vi "PicoScope6000aSetupStreaming.vi"(0 "handle in":i16=16384, 1 "Streaming Acquisition Settings":T4={"preTriggerSamples"=0, "postTriggerSamples"=1000000, "Requested sampleInterval"=1.0, "sampleIntervalTimeUnits"=3} {"sampleIntervalTimeUnits" items=["femtoseconds", "picoseconds", "nanoseconds", "microseconds", "millseconds", "seconds"]; "postTriggerSamples" format="%_6p"; "preTriggerSamples" format="%_6p"}, 2 "Buffer and Transfer Settings":T3={"startIndex"=0, "Samples"=1000000, "Down Sample Ratio"=1, "Down-Sample Mode"=2147483648} {"Down-Sample Mode" items=["None"=2147483648, "Aggregate"=1, "Decimate"=2, "Average"=4]; "Down Sample Ratio" step=1; "Samples" format="%_6p"}, 3 "enabled array":i16[](array[numeric])=[1, 1, 0, 0, 0, 0, 0, 0, 0, 0], 7 "Data Pointers In":T1, 9 "Number of Buffers":i32=1, 11 "error in (no error)":errorcluster) -> (4 "handle out":i16=16384, 8 "Data Pointers":T1, 13 "Actual sampleInterval":T2, 15 "error out":errorcluster)   [LabVIEW 2016]
doc: "Setup streaming Pico data buffers and first calls to ps6000aSetDataDataBuffer"
uses:
  ps6000a.dll
  shared/PicoBuffers.ctl
panel:
  in  "Dummy enabled array":i16[](array[numeric])=[1, 1, 0, 0, 0, 0, 0, 0, 0, 0]
  out "Actionflag":bool=TRUE
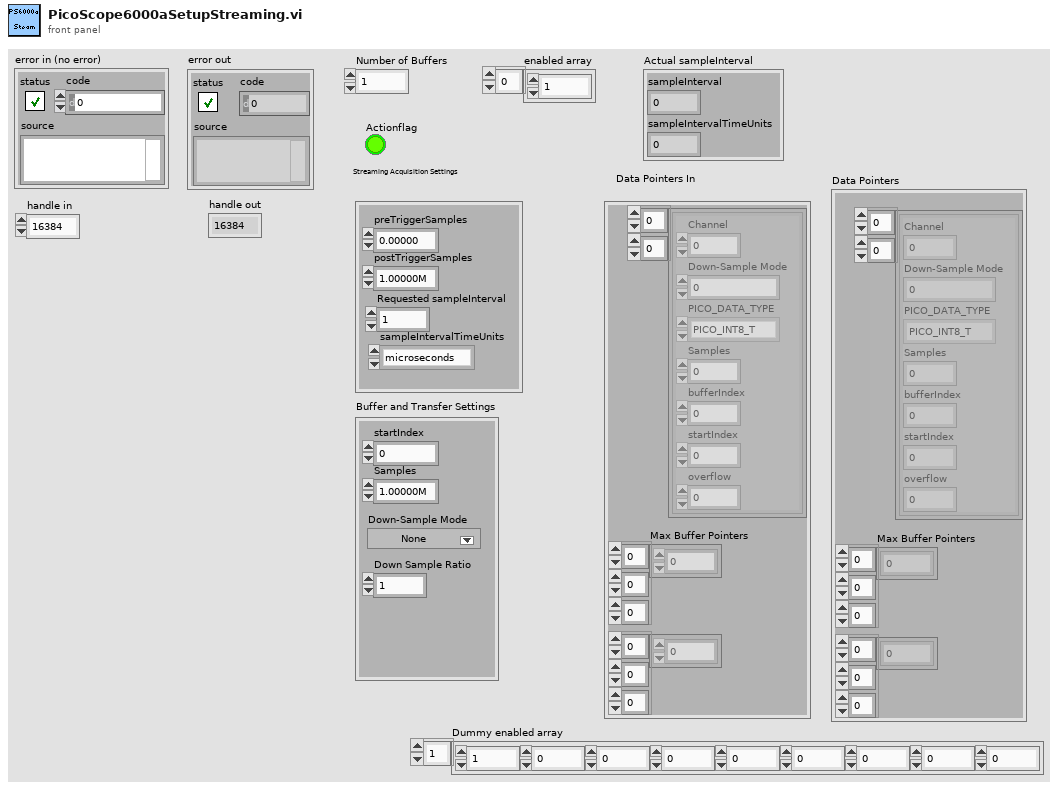
[diagram p1: front panel]
types:
  T1 = typedef "PicoBuffers.ctl" = cluster{"Max Buffer Pointers":u64[][][], "Min Buffer Pointers":u64[][][], "StreamingDataInfo":cluster{"Channel":u32, "Down-Sample Mode":u32, "PICO_DATA_TYPE":enum32{"PICO_INT8_T", "PICO_INT16_T", "PICO_INT32_T", "PICO_UINT32_T", "PICO_INT64_T", ""}, "Samples":i32, "bufferIndex":u64, "startIndex":i32, "overflow":i16}[][]}
  T2 = cluster{"sampleInterval":dbl, "sampleIntervalTimeUnits":u32}
  T3 = cluster{"startIndex":u64, "Samples":u64, "Down Sample Ratio":u64, "Down-Sample Mode":u32}
  T4 = cluster{"preTriggerSamples":u64, "postTriggerSamples":u64, "Requested sampleInterval":dbl, "sampleIntervalTimeUnits":u32}
  T5 = enum32{"PICO_INT8_T", "PICO_INT16_T", "PICO_INT32_T", "PICO_UINT32_T", "PICO_INT64_T", ""}
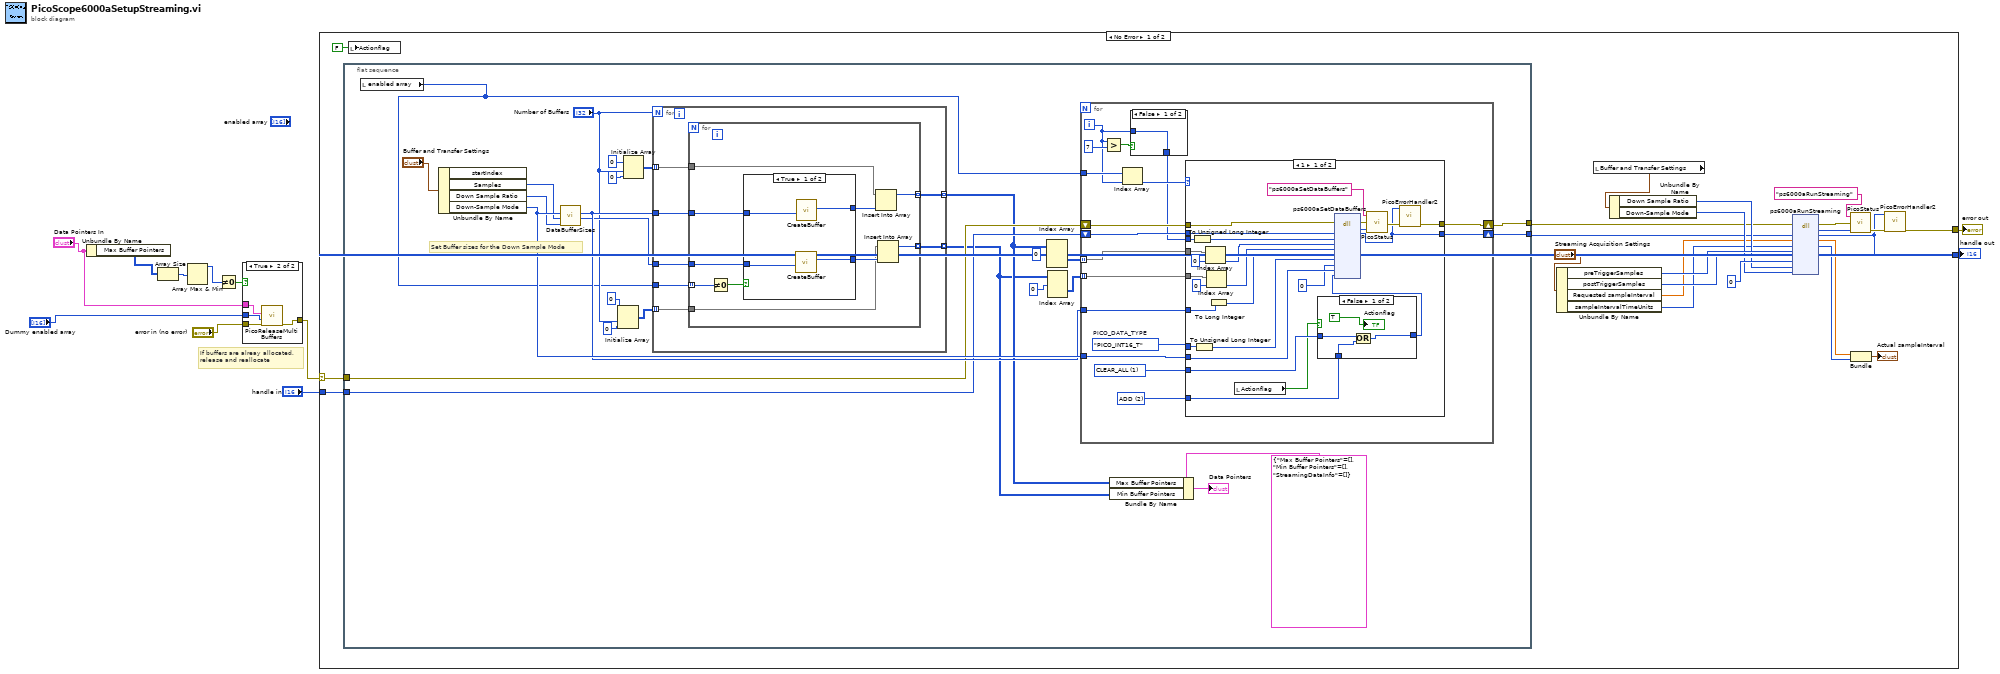
[diagram p0: block diagram]
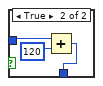
[diagram p3: hidden frame]
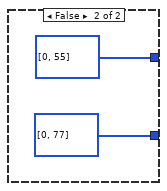
[diagram p6: hidden frame]
diagram:
  # "If buffers are alreay allocated,\nrelease and reallocate"
  n1 = Unbundle By Name("Data Pointers In") -> ("Max Buffer Pointers"=w3:u64[][][])
  n2 = Array Size(array=w3) -> (size(s)=w7:i32[])
  n3 = Array Max & Min(array=w7) -> (max value=w6:i32)  [unwired: 3 out]
  n4 = Not Equal To 0?(x=w6) -> (x != 0?=w8:bool)
  n5 = case shown="True" w8 {
    tunnel: "error in (no error)" -> [w12 w16]
    tunnel: [w12 w15] -> w4
    tunnel: "Dummy enabled array" -> [_ w14]
    tunnel: "Data Pointers In" -> [_ w13]
    frame False {
    }
    frame True {
      n6 = call "PicoReleaseMultiBuffers.vi"("error in (no error)"=w16, "Enabled array"=w14, "Data Pointers"=w13) -> ("error out"=w15:errorcluster)  [unwired: 8 in]
    }
  }
  n7 = case shown="No Error" w4 {
    selector: w4 -> [w28 w143]
    tunnel: "handle in" -> [w27 w144]
    tunnel: [w20 w144] -> w10
    tunnel: [w21 w143] -> w9
    frame No Error {
      n8 = flat-sequence {
        tunnel: w28 -> [w48]
        tunnel: w27 -> [w49]
        tunnel: [w50] -> w26
        tunnel: [w45] -> w25
        frame #0 {
          # "Set Buffer sizes for the Down Sample Mode"
          n9 = local read "enabled array"() -> (w40:i16[])
          n10 = Unbundle By Name("Buffer and Transfer Settings") -> ("Samples"=w58:u64, "Down Sample Ratio"=w57:u64, "Down-Sample Mode"=w59:u32)  [unwired: 1 out]
          n11 = call "DataBufferSizes.vi"("Down Sample Ratio"=w57, "Number of Samples"=w58, "Down-Sample Mode"=w59) -> ("min Buffer Size"=w55:i32, "Max Buffer Size"=w56:i32)  [unwired: 7 in]
          n12 = Initialize Array(u64 0 ("element"), "Number of Buffers", 0 ("dimension size")) -> (w52:u64[][])
          n13 = Initialize Array(u64 0 ("element"), "Number of Buffers", 0 ("dimension size")) -> (w60:u64[][])
          n14 = for {
            N: "Number of Buffers" -> [_]
            tunnel: w40 -> [w125]
            tunnel: w56 -> [w126]
            tunnel: w55 -> [w124]
            tunnel: [w123] -> w44 mode=indexing
            tunnel: w60 -> [w122] mode=indexing
            tunnel: w52 -> [w121] mode=indexing
            tunnel: [w120] -> w43 mode=indexing
            n15 = for {
              tunnel: w126 -> [w136]
              tunnel: w125 -> [w134] mode=indexing
              tunnel: w124 -> [w133]
              tunnel: [w131] -> w123 mode=indexing
              tunnel: w122 -> [w130]
              tunnel: w121 -> [w128]
              tunnel: [w127] -> w120 mode=indexing
              n16 = Not Equal To 0?(x=w134) -> (x != 0?=w135:bool)
              n17 = case shown="True" w135 {
                tunnel: w136 -> [w139 _]
                tunnel: w133 -> [w140 _]
                tunnel: [w138 u64[] [0, 55]] -> w132
                tunnel: [w137 u64[] [0, 77]] -> w129
                frame True {
                  n18 = call "CreateBuffer.vi"("Buffer size"=w140) -> ("Pointer and BufferSize"=w137:u64[])  [unwired: 9 in, 1 out]
                  n19 = call "CreateBuffer.vi"("Buffer size"=w139) -> ("Pointer and BufferSize"=w138:u64[])  [unwired: 9 in, 1 out]
                }
                frame False {
                }
              }
              n20 = Insert Into Array(array=w130, new element=w132) -> (w131:u64[])  [unwired: 1 in]
              n21 = Insert Into Array(array=w128, new element=w129) -> (w127:u64[])  [unwired: 1 in]
            }
          }
          n22 = Index Array(array=w44, index (dim 0)=0 ("index")) -> (element=w63:u64[][])  [unwired: 2 in]
          n23 = Index Array(array=w43, index (dim 0)=0 ("index")) -> (element=w46:u64[][])  [unwired: 2 in]
          n24 = for {
            tunnel: w59 -> [w82]
            tunnel: w56 -> [w74]
            tunnel: w40 -> [w79]
            tunnel: w63 -> [w73] mode=indexing
            shift-right: [w72] -> w50
            shift-left: w48 -> [w81]
            tunnel: w46 -> [w67] mode=indexing
            shift-right: [w66] -> w45
            shift-left: w49 -> [w80]
            i -> [w71]
            w68 = T5."PICO_INT16_T"  # PICO_DATA_TYPE
            w69 = u32 1 items=["NONE"=0, "CLEAR_ALL"=1, "ADD"=2, "CLEAR_THIS_DATA_BUFFER"=4096, "CLEAR_WAVEFORM_DATA_BUFFERS"=8192, "CLEAR_WAVEFORM_READ_DATA_BUFFERS"=16384] ("PicoAction 1")
            w70 = u32 2 items=["NONE"=0, "CLEAR_ALL"=1, "ADD"=2, "CLEAR_THIS_DATA_BUFFER"=4096, "CLEAR_WAVEFORM_DATA_BUFFERS"=8192, "CLEAR_WAVEFORM_READ_DATA_BUFFERS"=16384] ("PicoAction 2")
            n25 = Greater?(x=w71, y=7) -> (0:w76:bool)
            n26 = Index Array(array=w79, index=w71) -> (element=w78:i16)
            n27 = case shown="False" w76 {
              tunnel: [w83 w84] -> w75
              tunnel: w71 -> [w83 w86]
              frame False {
              }
              frame True {
                n28 = Add(x=w86, y=120) -> (x+y=w84:i32)
              }
            }
            n29 = case shown="1" w78 {
              tunnel: w75 -> [w101 _]
              tunnel: w81 -> [w112 w119]
              tunnel: w80 -> [w109 w118]
              tunnel: w82 -> [w106 _]
              tunnel: w68 -> [w91 _]
              tunnel: w69 -> [w96 _]
              tunnel: [w105 w119] -> w72
              tunnel: [w104 w118] -> w66
              tunnel: w74 -> [w103 _]
              tunnel: w73 -> [w97 _]
              tunnel: w70 -> [w95 _]
              tunnel: w67 -> [w87 _]
              frame 1 {
                n30 = To Unsigned Long Integer(number=w101) -> (unsigned 32bit integer=w100:u32)
                n31 = To Unsigned Long Integer(number=w91) -> (unsigned 32bit integer=w92:u32)
                n32 = Index Array(array=w97, index=0) -> (element=w98:u64)
                n33 = Index Array(array=w87, index=0) -> (element=w88:u64)
                n34 = To Long Integer(number=w103) -> (32bit integer=w102:i32)
                n35 = local read "Actionflag"() -> (w93:bool)
                n36 = case shown="False" w93 {
                  tunnel: w96 -> [w116 _]
                  tunnel: w95 -> [w115 w117]
                  tunnel: [w114 w117] -> w94
                  frame False {
                    n37 = Or(x=w116, y=w115) -> (x .or. y?=w114:u32)
                    "Actionflag" <- TRUE ("Actionflag")
                  }
                  frame True {
                  }
                }
                n38 = dll-call lib="ps6000a.dll" fn="ps6000aSetDataBuffers" ("ps3000.dll:_ps3000_open_unit@0")(error in=w112, "handle"=w109, "channel"=w100, "bufferMax"=w98, "bufferMin"=w88, "nSamples"=w102, "dataType"=w92, "waveform"=u64 0, "downSampleRatioMode"=w106, "action"=w94) -> (error out=w111:errorcluster, "PICO_STATUS"=w110:u32, "handle"=w104:i16)  [unwired: 10 in, 1 out]
                n39 = call "PicoStatus.vi"("PICO STATUS"=w110, "error in"=w111, "source"="ps6000aSetDataBuffers") -> ("error out"=w107:errorcluster)
                n40 = call "PicoErrorHandler2.vi"("error in (no error)"=w107, "handle In"=w104) -> ("error out"=w105:errorcluster)  [unwired: 9 in]
              }
              frame 0, Default {
              }
            }
          }
          n41 = Bundle By Name(cluster=T1 {"Max Buffer Pointers"=[], "Min Buffer Pointers"=[], "StreamingDataInfo"=[]} ("Data Pointers"), "Max Buffer Pointers"=w44, "Min Buffer Pointers"=w43) -> (→"Data Pointers":T1)
        }
      }
      n42 = local write "Actionflag"(FALSE ("Actionflag")) -> ()
      n43 = Unbundle By Name("Streaming Acquisition Settings") -> ("preTriggerSamples"=w33:u64, "postTriggerSamples"=w32:u64, "Requested sampleInterval"=w24:dbl, "sampleIntervalTimeUnits"=w23:u32)
      n44 = local read "Buffer and Transfer Settings"() -> (w31:T3)
      n45 = Unbundle By Name(w31) -> ("Down Sample Ratio"=w30:u64, "Down-Sample Mode"=w29:u32)
      n46 = dll-call lib="ps6000a.dll" fn="ps6000aRunStreaming" ("ps3000.dll:_ps3000_open_unit@0")(error in=w26, "handle"=w25, "sampleInterval"=w24, "sampleIntervalTimeUnits"=w23, "maxPreTriggerSamples"=w33, "maxPostPreTriggerSamples"=w32, "autoStop"=i16 0, "downSampleRatio"=w30, "downSampleRatioMode"=w29) -> (error out=w38:errorcluster, "PICO_STATUS"=w37:u32, "handle"=w20:i16, "sampleInterval"=w19:dbl, "sampleIntervalTimeUnits"=w18:u32)  [unwired: 7 in, 1 out]
      n47 = call "PicoStatus.vi"("PICO STATUS"=w37, "error in"=w38, "source"="ps6000aRunStreaming") -> ("error out"=w39:errorcluster)
      n48 = Bundle("sampleInterval"=w19, "sampleIntervalTimeUnits"=w18) -> (→"Actual sampleInterval":T2)  [unwired: 1 in]
      n49 = call "PicoErrorHandler2.vi"("error in (no error)"=w39, "handle In"=w20) -> ("error out"=w21:errorcluster)  [unwired: 9 in]
    }
    frame Error {
    }
  }
  "handle out" <- w10
  "error out" <- w9
